vi "LS372Monitor.vi"() -> ()   [LabVIEW 2019]
uses:
  Utility/LS372/LS372-Cluster.ctl
  Instrument_Setup.vi
  Global/Global Variables/Data_Display_global.vi
  Global/Global Variables/global.vi
  Equipment/Lake Shore 372/Lake Shore 372.lvlib
panel:
  out "Tsweeps Running":bool
  out "LS372-Cluster":T1 {"MC Thermometer" items=["Speer 9905", "ROX U02453"]}
  in  "Stopp":bool
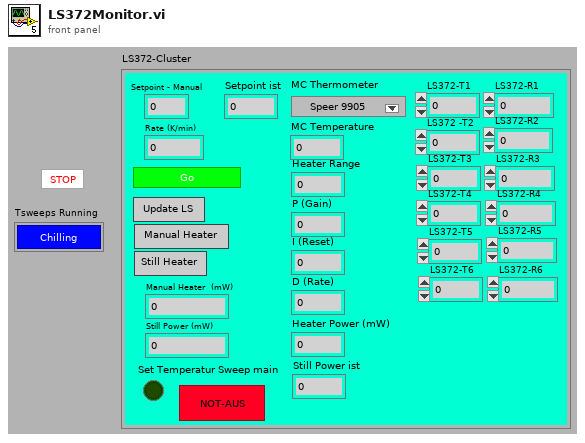
[diagram p1: front panel]
types:
  T1 = typedef "LS372-Cluster.ctl" = cluster{"Activate Tsweep":bool, "Setpoint - Manual":dbl, "Rate (K/min)":dbl, "Update Lakeshores":bool, "Still Heater":bool, "Still Power (mW)":dbl, "Manual Heater":bool, "Manual Heater  (mW) ":dbl, "Heater Range":dbl, "P (Gain)":dbl, "I (Reset)":dbl, "D (Rate)":dbl, "Heater Power (mW)":dbl, "MC Thermometer":u16, "MC Temperature":dbl, "LS372-T1":dbl, "LS372 -T2":dbl, "LS372-R1 ":dbl, "LS372-R2":dbl, "LS372-T3":dbl, "LS372-T4":dbl, "LS372-R3 ":dbl, "LS372-R4 \n\n\n\n":dbl, "LS372-T5":dbl, "LS372-T6":dbl, "LS372-R5":dbl, "LS372-R6 ":dbl, "Still Power ist":dbl, "Set Temperatur Sweep main":bool, "Setpoint ist":dbl, "Disable Heater":bool}
  T2 = typedef "Ls372-Control.ctl" = cluster{"Activate Tsweep":bool, "Setpoint - Manual":dbl, "Rate (K/min)":dbl, "Update Lakeshores":bool, "Still Heater":bool, "Still Power (mW)":dbl, "Manual Heater":bool, "Manual Heater  (mW) ":dbl, "MC Thermometer":u16, "Set Temperature Sweeep main":bool, "Disable Heater":bool}
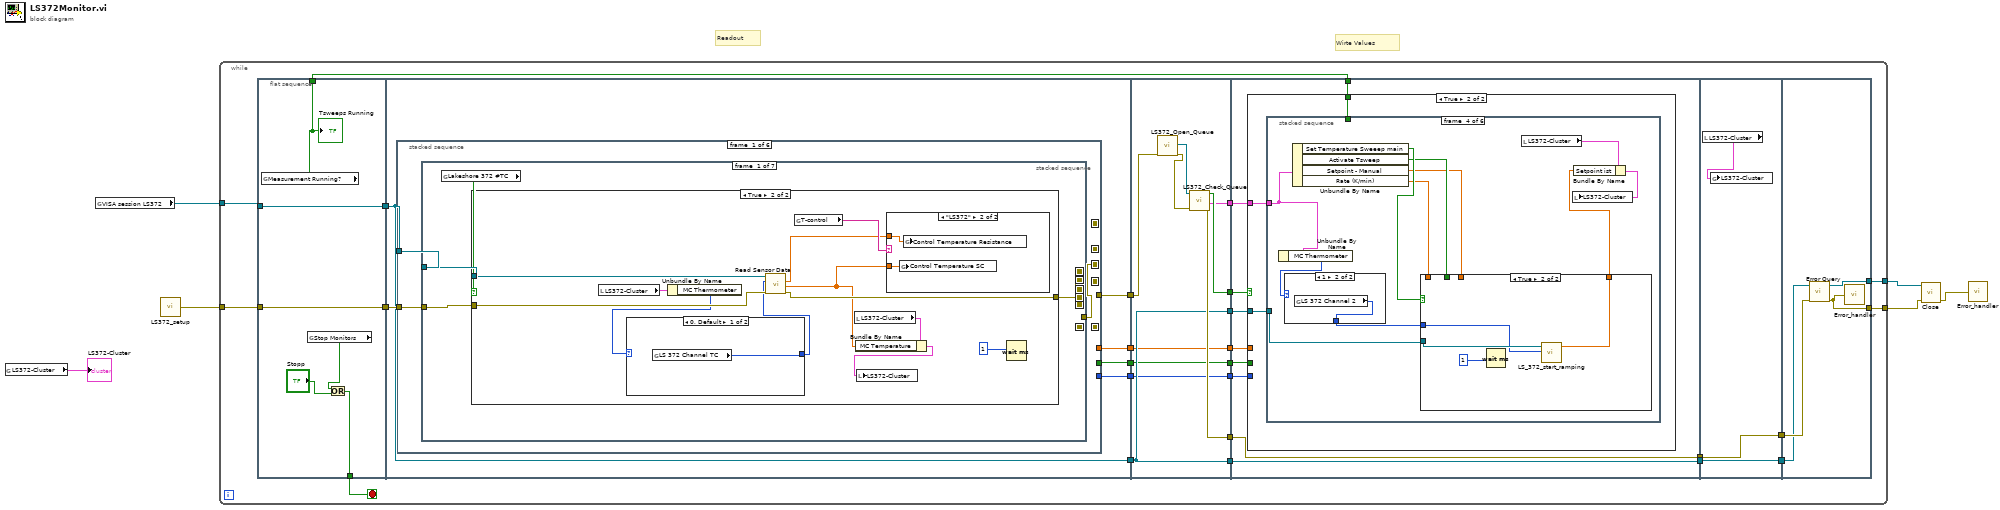
[diagram p0: block diagram]
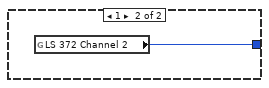
[diagram p3: hidden frame]
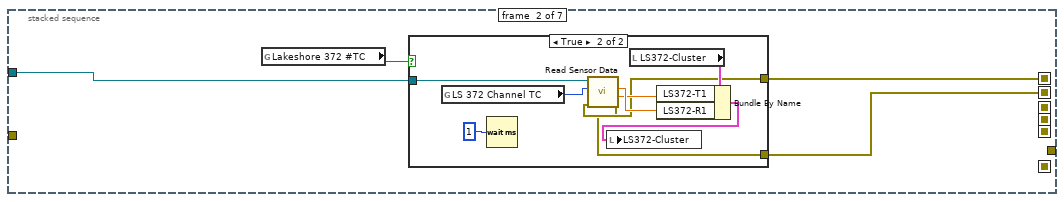
[diagram p5: hidden frame]
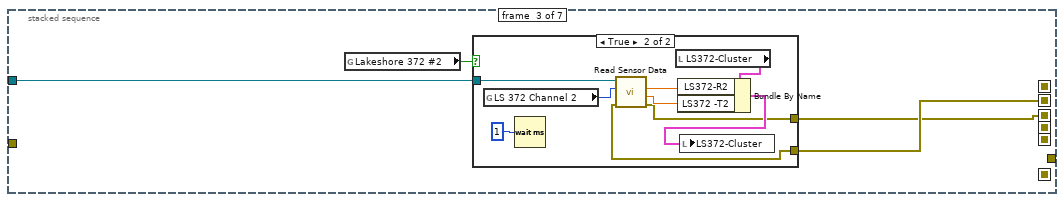
[diagram p7: hidden frame]
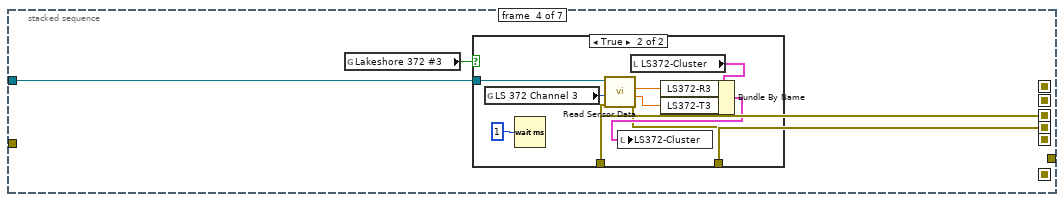
[diagram p9: hidden frame]
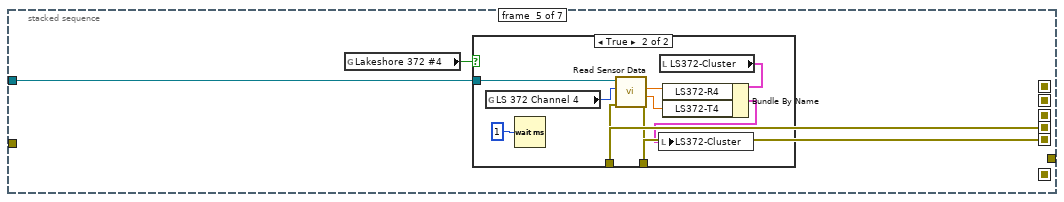
[diagram p11: hidden frame]
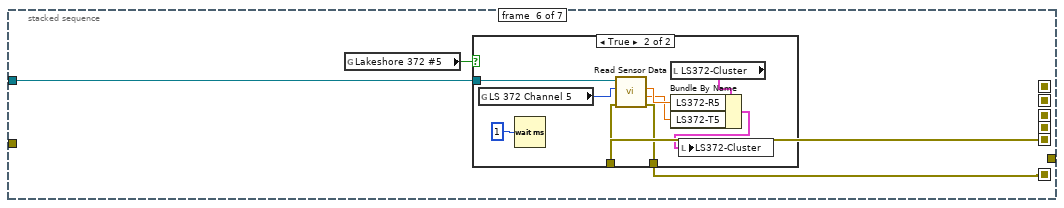
[diagram p13: hidden frame]
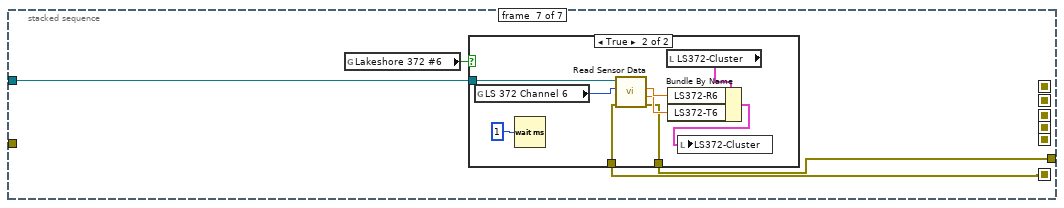
[diagram p15: hidden frame]
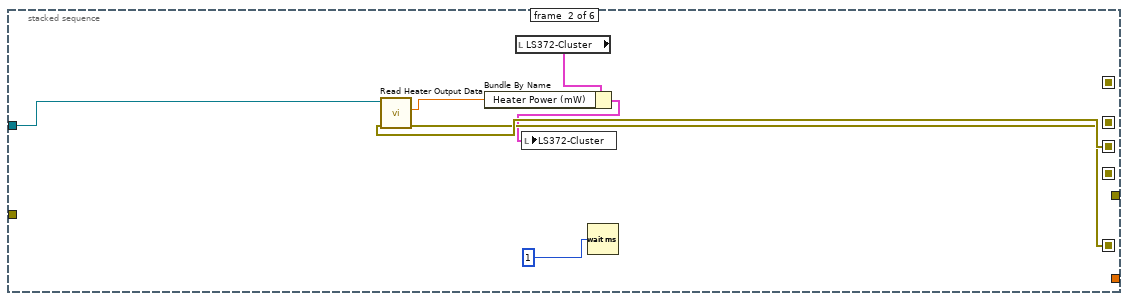
[diagram p17: hidden frame]
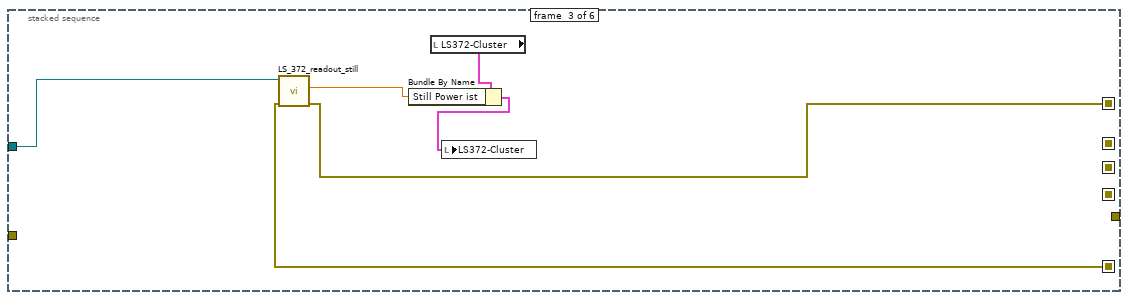
[diagram p18: hidden frame]
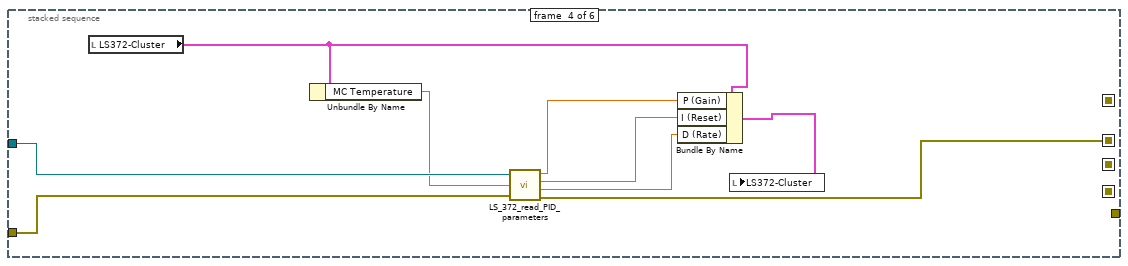
[diagram p19: hidden frame]
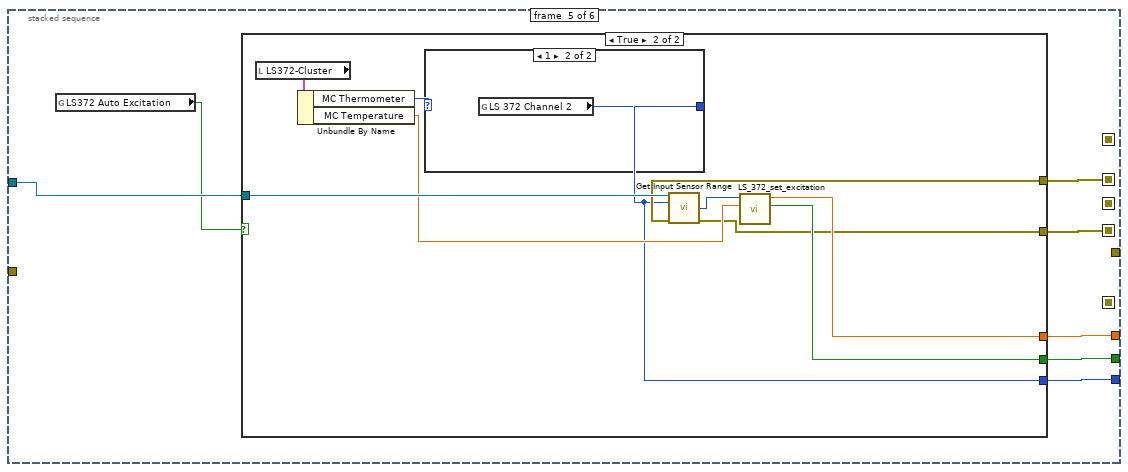
[diagram p20: hidden frame]
diagram:
  # "Wirte Values"
  # "Readout"
  n1 = global read "Data_Display_global.vi" "LS372-Cluster"() -> (→"LS372-Cluster":T1)
  n2 = global read "Instrument_Setup.vi" "VISA session LS372"() -> (w6:refnum<visa-resource-name>)
  n3 = call "LS372_setup.vi"() -> ("error out"=w4:errorcluster)
  n4 = while {
    tunnel: w6 -> [w31]
    tunnel: w4 -> [w25]
    tunnel: [w14] -> w3
    tunnel: [w13] -> w2
    stop <- w29 stop-if-true
    n5 = flat-sequence {
      tunnel: w31 -> [w35]
      tunnel: [w35] -> w30
      tunnel: [w32] -> w29
      tunnel: w25 -> [w34]
      tunnel: [w34] -> w24
      tunnel: [w33] -> w21
      tunnel: w30 -> [w41]
      tunnel: [w42] -> w28
      tunnel: w24 -> [w43]
      tunnel: [w41] -> w23
      tunnel: [w40] -> w11
      tunnel: [w39] -> w9
      tunnel: [w38] -> w7
      tunnel: w28 -> [w212]
      tunnel: [w209] -> w27
      tunnel: [w208] -> w26
      tunnel: w23 -> [w206]
      tunnel: [w206] -> w22
      tunnel: [w207] -> w19
      tunnel: [w206] -> w15
      tunnel: [w205] -> w12
      tunnel: w11 -> [w205]
      tunnel: [w204] -> w10
      tunnel: w9 -> [w204]
      tunnel: [w203] -> w8
      tunnel: w7 -> [w203]
      tunnel: w27 -> [w221]
      tunnel: w26 -> [w220]
      tunnel: w22 -> [w219]
      tunnel: w21 -> [w218]
      tunnel: [w217] -> w20
      tunnel: w19 -> [w217]
      tunnel: [w216] -> w16
      tunnel: w15 -> [w216]
      tunnel: w12 -> [w215]
      tunnel: w10 -> [w214]
      tunnel: w8 -> [w213]
      tunnel: w20 -> [w322]
      tunnel: [w322] -> w18
      tunnel: [w321] -> w17
      tunnel: w16 -> [w321]
      tunnel: w18 -> [w327]
      tunnel: w17 -> [w326]
      tunnel: [w325] -> w14
      tunnel: [w324] -> w13
      frame #0 {
        n6 = global read "global.vi" "Measurement Running?"() -> (w33:bool)
        "Tsweeps Running" <- w33
        n7 = global read "Data_Display_global.vi" "Stop Monitors"() -> (w36:bool)
        n8 = Or(x=w36, y="Stopp") -> (x .or. y?=w32:bool)
      }
      frame #1 {
        n9 = stacked-sequence {
          seq-local: [w44 _ _ _ _ _] -> [_ w156 _ _ _ _]
          seq-local: [_ w155 _ _ _ _] -> [_ _ w163 _ _ _]
          seq-local: [_ _ w162 _ _ _] -> [_ _ _ _ _ _]
          seq-local: [_ _ _ w171 _ _] -> [_ _ _ _ w179 _]
          seq-local: [_ _ _ _ w175 _] -> [_ _ _ _ _ w201]
          tunnel: w41 -> [w46 w158 w164 w173 w180 w202]
          tunnel: w43 -> [w45 _ _ w172 _ _]
          tunnel: [_ _ _ _ _ w200] -> w42
          tunnel: [_ _ _ _ w178 _] -> w40
          tunnel: [_ _ _ _ w177 _] -> w39
          tunnel: [_ _ _ _ w176 _] -> w38
          frame #0 {
            n10 = stacked-sequence {
              seq-local: [w48 _ _ _ _ _ _] -> [_ w69 _ _ _ _ _]
              seq-local: [_ w68 _ _ _ _ _] -> [_ _ w83 _ _ _ _]
              seq-local: [_ _ w82 _ _ _ _] -> [_ _ _ w97 _ _ _]
              seq-local: [_ _ _ w96 _ _ _] -> [_ _ _ _ w111 _ _]
              seq-local: [_ _ _ _ w110 _ _] -> [_ _ _ _ _ w125 _]
              seq-local: [_ _ _ _ _ w124 _] -> [_ _ _ _ _ _ w139]
              tunnel: w46 -> [w50 w70 w84 w98 w112 w126 w140]
              tunnel: w45 -> [w47 _ _ _ _ _ _]
              tunnel: [_ _ _ _ _ _ w138] -> w44
              frame #0 {
                n11 = global read "Instrument_Setup.vi" "Lakeshore 372 #TC"() -> (w49:bool)
                n12 = case shown="True" w49 {
                  tunnel: w50 -> [_ w63]
                  tunnel: [w51 w62] -> w48
                  tunnel: w47 -> [w51 w61]
                  frame False {
                  }
                  frame True {
                    n13 = local read "LS372-Cluster"() -> (w55:T1)
                    n14 = Unbundle By Name(w55) -> ("MC Thermometer"=w54:u16)
                    n15 = case shown="0, Default" w54 {
                      tunnel: [w64 w65] -> w53
                      frame 0, Default {
                        n16 = global read "Instrument_Setup.vi" "LS 372 Channel TC"() -> (w64:u16)
                      }
                      frame 1 {
                        n17 = global read "Instrument_Setup.vi" "LS 372 Channel 2"() -> (w65:u16)
                      }
                    }
                    n18 = call "Read Sensor Data.vi"("error in (no error)"=w61, "Channel (1:1)"=w53, "VISA resource name"=w63) -> ("error out"=w62:errorcluster, "Kelvin Reading"=w57:dbl, "Resistance Reading"=w59:dbl)  [unwired: 3 in, 3 out]
                    n19 = global read "Instrument_Setup.vi" "T-control"() -> (w60:string)
                    n20 = local read "LS372-Cluster"() -> (w58:T1)
                    n21 = Bundle By Name(cluster=w58, "MC Temperature"=w57) -> (w56:T1)
                    n22 = local write "LS372-Cluster"(w56) -> ()
                    n23 = case shown="\"LS372\"" w60 {
                      tunnel: w59 -> [_ w67]
                      tunnel: w57 -> [_ w66]
                      frame "None", Default {
                      }
                      frame "LS372" {
                        n24 = global write "Data_Display_global.vi" "Control Temperature SC"(w66) -> ()
                        n25 = global write "Data_Display_global.vi" "Control Temperature Resistance"(w67) -> ()
                      }
                    }
                    n26 = Wait (ms)(milliseconds to wait=1) -> ()  [unwired: 1 out]
                  }
                }
              }
              frame #1 {
                n27 = global read "Instrument_Setup.vi" "Lakeshore 372 #TC"() -> (w71:bool)
                n28 = case shown="True" w71 {
                  tunnel: w70 -> [_ w80]
                  tunnel: w69 -> [w72 w74]
                  tunnel: [w72 w73] -> w68
                  frame False {
                  }
                  frame True {
                    n29 = global read "Instrument_Setup.vi" "LS 372 Channel TC"() -> (w79:u16)
                    n30 = Wait (ms)(milliseconds to wait=1) -> ()  [unwired: 1 out]
                    n31 = call "Read Sensor Data.vi"("error in (no error)"=w74, "Channel (1:1)"=w79, "VISA resource name"=w80) -> ("error out"=w73:errorcluster, "Kelvin Reading"=w75:dbl, "Resistance Reading"=w76:dbl)  [unwired: 3 in, 3 out]
                    n32 = local read "LS372-Cluster"() -> (w78:T1)
                    n33 = Bundle By Name(cluster=w78, "LS372-T1"=w75, "LS372-R1"=w76) -> (w77:T1)
                    n34 = local write "LS372-Cluster"(w77) -> ()
                  }
                }
              }
              frame #2 {
                n35 = global read "Instrument_Setup.vi" "Lakeshore 372 #2"() -> (w85:bool)
                n36 = case shown="True" w85 {
                  tunnel: w84 -> [_ w94]
                  tunnel: w83 -> [w86 w88]
                  tunnel: [w86 w87] -> w82
                  frame False {
                  }
                  frame True {
                    n37 = global read "Instrument_Setup.vi" "LS 372 Channel 2"() -> (w93:u16)
                    n38 = Wait (ms)(milliseconds to wait=1) -> ()  [unwired: 1 out]
                    n39 = call "Read Sensor Data.vi"("error in (no error)"=w88, "Channel (1:1)"=w93, "VISA resource name"=w94) -> ("error out"=w87:errorcluster, "Kelvin Reading"=w89:dbl, "Resistance Reading"=w90:dbl)  [unwired: 3 in, 3 out]
                    n40 = local read "LS372-Cluster"() -> (w92:T1)
                    n41 = Bundle By Name(cluster=w92, "LS372-R2"=w90, "LS372 -T2"=w89) -> (w91:T1)
                    n42 = local write "LS372-Cluster"(w91) -> ()
                  }
                }
              }
              frame #3 {
                n43 = global read "Instrument_Setup.vi" "Lakeshore 372 #3"() -> (w99:bool)
                n44 = case shown="True" w99 {
                  tunnel: w98 -> [_ w108]
                  tunnel: w97 -> [w100 w102]
                  tunnel: [w100 w101] -> w96
                  frame False {
                  }
                  frame True {
                    n45 = global read "Instrument_Setup.vi" "LS 372 Channel 3"() -> (w107:u16)
                    n46 = Wait (ms)(milliseconds to wait=1) -> ()  [unwired: 1 out]
                    n47 = call "Read Sensor Data.vi"("error in (no error)"=w102, "Channel (1:1)"=w107, "VISA resource name"=w108) -> ("error out"=w101:errorcluster, "Kelvin Reading"=w103:dbl, "Resistance Reading"=w104:dbl)  [unwired: 3 in, 3 out]
                    n48 = local read "LS372-Cluster"() -> (w106:T1)
                    n49 = Bundle By Name(cluster=w106, "LS372-R3"=w104, "LS372-T3"=w103) -> (w105:T1)
                    n50 = local write "LS372-Cluster"(w105) -> ()
                  }
                }
              }
              frame #4 {
                n51 = global read "Instrument_Setup.vi" "Lakeshore 372 #4"() -> (w113:bool)
                n52 = case shown="True" w113 {
                  tunnel: w112 -> [_ w122]
                  tunnel: w111 -> [w114 w116]
                  tunnel: [w114 w115] -> w110
                  frame False {
                  }
                  frame True {
                    n53 = global read "Instrument_Setup.vi" "LS 372 Channel 4"() -> (w121:u16)
                    n54 = Wait (ms)(milliseconds to wait=1) -> ()  [unwired: 1 out]
                    n55 = call "Read Sensor Data.vi"("error in (no error)"=w116, "Channel (1:1)"=w121, "VISA resource name"=w122) -> ("error out"=w115:errorcluster, "Kelvin Reading"=w117:dbl, "Resistance Reading"=w118:dbl)  [unwired: 3 in, 3 out]
                    n56 = local read "LS372-Cluster"() -> (w120:T1)
                    n57 = Bundle By Name(cluster=w120, "LS372-R4"=w118, "LS372-T4"=w117) -> (w119:T1)
                    n58 = local write "LS372-Cluster"(w119) -> ()
                  }
                }
              }
              frame #5 {
                n59 = global read "Instrument_Setup.vi" "Lakeshore 372 #5"() -> (w127:bool)
                n60 = case shown="True" w127 {
                  tunnel: w126 -> [_ w136]
                  tunnel: w125 -> [w128 w130]
                  tunnel: [w128 w129] -> w124
                  frame False {
                  }
                  frame True {
                    n61 = global read "Instrument_Setup.vi" "LS 372 Channel 5"() -> (w135:u16)
                    n62 = Wait (ms)(milliseconds to wait=1) -> ()  [unwired: 1 out]
                    n63 = call "Read Sensor Data.vi"("error in (no error)"=w130, "Channel (1:1)"=w135, "VISA resource name"=w136) -> ("error out"=w129:errorcluster, "Kelvin Reading"=w131:dbl, "Resistance Reading"=w132:dbl)  [unwired: 3 in, 3 out]
                    n64 = local read "LS372-Cluster"() -> (w134:T1)
                    n65 = Bundle By Name(cluster=w134, "LS372-R5"=w132, "LS372-T5"=w131) -> (w133:T1)
                    n66 = local write "LS372-Cluster"(w133) -> ()
                  }
                }
              }
              frame #6 {
                n67 = global read "Instrument_Setup.vi" "Lakeshore 372 #6"() -> (w141:bool)
                n68 = case shown="True" w141 {
                  tunnel: w140 -> [_ w150]
                  tunnel: w139 -> [w142 w144]
                  tunnel: [w142 w143] -> w138
                  frame False {
                  }
                  frame True {
                    n69 = global read "Instrument_Setup.vi" "LS 372 Channel 6"() -> (w149:u16)
                    n70 = Wait (ms)(milliseconds to wait=1) -> ()  [unwired: 1 out]
                    n71 = call "Read Sensor Data.vi"("error in (no error)"=w144, "Channel (1:1)"=w149, "VISA resource name"=w150) -> ("error out"=w143:errorcluster, "Kelvin Reading"=w145:dbl, "Resistance Reading"=w146:dbl)  [unwired: 3 in, 3 out]
                    n72 = local read "LS372-Cluster"() -> (w148:T1)
                    n73 = Bundle By Name(cluster=w148, "LS372-R6"=w146, "LS372-T6"=w145) -> (w147:T1)
                    n74 = local write "LS372-Cluster"(w147) -> ()
                  }
                }
              }
            }
          }
          frame #1 {
            n75 = call "Read Heater Output Data.vi"("error in (no error)"=w156, "VISA resource name"=w158) -> ("error out"=w155:errorcluster, "Heater Output"=w152:dbl)  [unwired: 7 in, 1 out]
            n76 = local read "LS372-Cluster"() -> (w154:T1)
            n77 = Bundle By Name(cluster=w154, "Heater Power (mW)"=w152) -> (w153:T1)
            n78 = local write "LS372-Cluster"(w153) -> ()
            n79 = Wait (ms)(milliseconds to wait=1) -> ()  [unwired: 1 out]
          }
          frame #2 {
            n80 = call "LS_372_readout_still.vi"("error in (no error)"=w163, "VISA-Ressourcenname (in)"=w164) -> ("error out"=w162:errorcluster, "Still Value"=w159:dbl)  [unwired: 3 in, 1 out]
            n81 = local read "LS372-Cluster"() -> (w161:T1)
            n82 = Bundle By Name(cluster=w161, "Still Power ist"=w159) -> (w160:T1)
            n83 = local write "LS372-Cluster"(w160) -> ()
          }
          frame #3 {
            n84 = local read "LS372-Cluster"() -> (w166:T1)
            n85 = Unbundle By Name(w166) -> ("MC Temperature"=w165:dbl)
            n86 = call "LS_372_read_PID_parameters.vi"("VISA-Ressourcenname (in)"=w173, "Temperature"=w165, "error in (no error)"=w172) -> ("Gain (P)"=w169:dbl, "Reset (I)"=w168:dbl, "Rate (D)"=w167:dbl, "error out"=w171:errorcluster)  [unwired: 1 out]
            n87 = Bundle By Name(cluster=w166, "P (Gain)"=w169, "I (Reset)"=w168, "D (Rate)"=w167) -> (w170:T1)
            n88 = local write "LS372-Cluster"(w170) -> ()
          }
          frame #4 {
            n89 = global read "Instrument_Setup.vi" "LS372 Auto Excitation"() -> (w174:bool)
            n90 = case shown="True" w174 {
              tunnel: w180 -> [_ w194]
              tunnel: w179 -> [w184 w193]
              tunnel: [5.0 w188] -> w178
              tunnel: [FALSE w187] -> w177
              tunnel: [1 w186] -> w176
              tunnel: [w184 w185] -> w175
              frame False {
              }
              frame True {
                n91 = local read "LS372-Cluster"() -> (w192:T1)
                n92 = Unbundle By Name(w192) -> ("MC Thermometer"=w191:u16, "MC Temperature"=w189:dbl)
                n93 = case shown="1" w191 {
                  tunnel: [w195 w196] -> w186
                  frame 0, Default {
                    n94 = global read "Instrument_Setup.vi" "LS 372 Channel TC"() -> (w195:u16)
                  }
                  frame 1 {
                    n95 = global read "Instrument_Setup.vi" "LS 372 Channel 2"() -> (w196:u16)
                  }
                }
                n96 = call "Get Input Sensor Range.vi"("VISA resource name"=w194, "Channel (1:1)"=w186, "error in (no error)"=w193) -> ("Excitation Range"=w190:u16, "error out"=w185:errorcluster)  [unwired: 5 in, 6 out]
                n97 = call "LS_372_set_excitation.vi"("Temperature"=w189, "LS_Excitation old"=w190) -> ("Change of Excitation?"=w187:bool, "LS_Excitation new"=w188:dbl)  [unwired: 4 in]
              }
            }
          }
          frame #5 {
            n98 = call "LS_372_read_heater_range.vi"("Error In"=w201, "VISA (in)"=w202) -> ("Error Out"=w200:errorcluster, "Numeric"=w197:dbl)  [unwired: 1 in, 1 out]
            n99 = local read "LS372-Cluster"() -> (w199:T1)
            n100 = Bundle By Name(cluster=w199, "Heater Range"=w197) -> (w198:T1)
            n101 = local write "LS372-Cluster"(w198) -> ()
          }
        }
      }
      frame #2 {
        n102 = call "LS372_Open_Queue.vi"("error in (no error)"=w212) -> ("error out"=w211:errorcluster, "queue out"=w210:refnum<queue>)  [unwired: 9 in]
        n103 = call "LS372_Check_Queue.vi"("error in (no error)"=w211, "queue"=w210) -> ("error out"=w207:errorcluster, "LS372-Control"=w208:T2, "New Entries?"=w209:bool)  [unwired: 6 in]
      }
      frame #3 {
        n104 = case shown="True" w221 {
          tunnel: w220 -> [_ w233]
          tunnel: w219 -> [w225 w232]
          tunnel: w218 -> [_ w231]
          tunnel: w215 -> [w224 _]
          tunnel: w214 -> [w222 _]
          tunnel: w213 -> [w223 _]
          frame False {
            n105 = case shown="True" w222 {
              tunnel: w225 -> [_ w230]
              tunnel: w224 -> [_ w229]
              tunnel: w223 -> [_ w228]
              frame False {
              }
              frame True {
                n106 = call "Configure Input Sensor Range.vi"("VISA resource name"=w230, "Channel (1)"=w228, "Excitation Range (5: 200 uV / 100 pA)"=w229, "Autorange (0: Autorange off)"=1, "Preferred Units (2: Ohms)"=1) -> ()  [unwired: 13 in, 2 out]
              }
            }
          }
          frame True {
            n107 = stacked-sequence {
              tunnel: w233 -> [w238 w255 w263 w268 w301 w320]
              tunnel: w232 -> [w236 w253 w256 w276 w302 _]
              tunnel: w231 -> [_ _ w262 _ _ _]
              frame #0 {
                n108 = Unbundle By Name(w238) -> ("Update Lakeshores"=w237:bool, "MC Thermometer"=w235:u16)
                n109 = case shown="1" w235 {
                  tunnel: [w239 w240] -> w234
                  frame 0, Default {
                    n110 = global read "Instrument_Setup.vi" "LS 372 Channel TC"() -> (w239:u16)
                  }
                  frame 1 {
                    n111 = global read "Instrument_Setup.vi" "LS 372 Channel 2"() -> (w240:u16)
                  }
                }
                n112 = case shown="True" w237 {
                  tunnel: w236 -> [_ w243]
                  tunnel: w234 -> [_ w241]
                  frame False {
                  }
                  frame True {
                    n113 = flat-sequence {
                      tunnel: [w246] -> w244
                      tunnel: w243 -> [w246]
                      tunnel: [w245] -> w242
                      tunnel: w241 -> [w245]
                      tunnel: w244 -> [w249]
                      tunnel: w242 -> [w248]
                      frame #0 {
                        n114 = call "LS372_setup.vi"() -> ()  [unwired: 1 out]
                        n115 = Wait (ms)(milliseconds to wait=50) -> ()  [unwired: 1 out]
                      }
                      frame #1 {
                        n116 = call "LS372_set_main_measuring_channel.vi"("VISA resource name"=w249, "Channel"=w248) -> ()  [unwired: 4 in, 1 out]
                      }
                    }
                  }
                }
              }
              frame #1 {
                # "Set Still Power"
                n117 = global read "Instrument_Setup.vi" "LS 372  Still Heater Resistance"() -> (w250:dbl)
                n118 = Unbundle By Name(w255) -> ("Still Heater"=w252:bool, "Still Power (mW)"=w251:dbl)
                n119 = call "LS_372_still_control.vi"("Still Resistance"=w250, "Still Power"=w251, "Still heater"=w252, "VISA-Ressourcenname"=w253) -> ()  [unwired: 4 in]
                n120 = Wait (ms)(milliseconds to wait=1) -> ()  [unwired: 1 out]
              }
              frame #2 {
                # "Set Heater Power manuel"
                n121 = Unbundle By Name(w263) -> ("Manual Heater  (mW)"=w258:dbl, "Manual Heater"=w260:bool)
                n122 = Not(x=w262) -> (.not. x?=w261:bool)
                n123 = And(x=w261, y=w260) -> (x .and. y?=w259:bool)
                n124 = case shown="True" w259 {
                  selector: w259 -> [_ w267]
                  tunnel: w258 -> [_ w266]
                  tunnel: w256 -> [_ w264]
                  frame False {
                  }
                  frame True {
                    n125 = global read "Instrument_Setup.vi" "LS 372 MC Heater Resistance"() -> (w265:dbl)
                    n126 = call "LS372_manual_heater_output.vi"("Heater Resistance"=w265, "Heater Power"=w266, "Manuel Heater"=w267, "VISA-Ressourcenname"=w264) -> ()  [unwired: 4 in]
                  }
                }
                n127 = Wait (ms)(milliseconds to wait=1) -> ()  [unwired: 1 out]
              }
              frame #3 {
                n128 = Unbundle By Name(w268) -> ("MC Thermometer"=w269:u16)
                n129 = case shown="1" w269 {
                  tunnel: [w279 w280] -> w270
                  frame 0, Default {
                    n130 = global read "Instrument_Setup.vi" "LS 372 Channel TC"() -> (w279:u16)
                  }
                  frame 1 {
                    n131 = global read "Instrument_Setup.vi" "LS 372 Channel 2"() -> (w280:u16)
                  }
                }
                n132 = Unbundle By Name(w268) -> ("Set Temperature Sweeep main"=w278:bool, "Activate Tsweep"=w277:bool, "Setpoint - Manual"=w272:dbl, "Rate (K/min)"=w271:dbl)
                n133 = case shown="True" w278 {
                  tunnel: w277 -> [w286 _]
                  tunnel: w276 -> [w282 w299]
                  tunnel: [w281 w298] -> w273
                  tunnel: w272 -> [w284 _]
                  tunnel: w271 -> [w285 _]
                  tunnel: w270 -> [w283 w297]
                  frame False {
                    n134 = case shown="True" w286 {
                      tunnel: w285 -> [_ w296]
                      tunnel: w284 -> [_ w293]
                      tunnel: w283 -> [_ w295]
                      tunnel: w282 -> [_ w294]
                      tunnel: [w287 w293] -> w281
                      frame False {
                        n135 = global read "global.vi" "Cerrent State"() -> (w290:i32)
                        n136 = Equal?(x=1, y=w290) -> (x = y?=w288:bool)
                        n137 = case shown="False" w288 {
                          tunnel: [w291 w292] -> w287
                          frame False {
                            n138 = global read "global.vi" "T final (K)"() -> (w291:dbl)
                          }
                          frame True {
                            n139 = global read "global.vi" "T init. (K)"() -> (w292:dbl)
                          }
                        }
                      }
                      frame True {
                        n140 = call "LS_372_manual_ramping.vi"("Setpoint"=w293, "Rate"=w296, "Channel"=w295, "VISA-Ressourcenname"=w294) -> ()  [unwired: 4 in]
                      }
                    }
                  }
                  frame True {
                    n141 = Wait (ms)(milliseconds to wait=1) -> ()  [unwired: 1 out]
                    n142 = call "LS_372_start_ramping.vi"("Channel"=w297, "VISA-Ressourcenname"=w299) -> ("Setpoint"=w298:dbl)  [unwired: 5 in]
                  }
                }
                n143 = local read "LS372-Cluster"() -> (w275:T1)
                n144 = Bundle By Name(cluster=w275, "Setpoint ist"=w273) -> (w274:T1)
                n145 = local write "LS372-Cluster"(w274) -> ()
              }
              frame #4 {
                n146 = Unbundle By Name(w301) -> ("Disable Heater"=w303:bool)
                n147 = case shown="True" w303 {
                  tunnel: w302 -> [_ w305]
                  tunnel: w301 -> [_ w304]
                  frame False {
                  }
                  frame True {
                    n148 = Unbundle By Name(w304) -> ("MC Thermometer"=w309:u16)
                    n149 = case shown="0, Default" w309 {
                      tunnel: [w312 w315] -> w306
                      tunnel: w305 -> [w311 w314]
                      frame 0, Default {
                        n150 = global read "Instrument_Setup.vi" "LS 372 Channel TC"() -> (w313:u16)
                        n151 = call "LS_372_disable_heater.vi"("Channel"=w313, "VISA-Ressourcenname"=w311) -> ("Setpoint ist"=w312:dbl)  [unwired: 5 in]
                      }
                      frame 1 {
                        n152 = global read "Instrument_Setup.vi" "LS 372 Channel 2"() -> (w316:u16)
                        n153 = call "LS_372_disable_heater.vi"("Channel"=w316, "VISA-Ressourcenname"=w314) -> ("Setpoint ist"=w315:dbl)  [unwired: 5 in]
                      }
                    }
                    n154 = local read "LS372-Cluster"() -> (w308:T1)
                    n155 = Bundle By Name(cluster=w308, "Setpoint ist"=w306) -> (w307:T1)
                    n156 = local write "LS372-Cluster"(w307) -> ()
                    n157 = Wait (ms)(milliseconds to wait=10) -> ()  [unwired: 1 out]
                  }
                }
              }
              frame #5 {
                n158 = Unbundle By Name(w320) -> ("MC Thermometer"=w318:u16)
                n159 = local read "LS372-Cluster"() -> (w319:T1)
                n160 = Bundle By Name(cluster=w319, "MC Thermometer"=w318) -> (w317:T1)
                n161 = local write "LS372-Cluster"(w317) -> ()
              }
            }
          }
        }
      }
      frame #4 {
        n162 = local read "LS372-Cluster"() -> (w323:T1)
        n163 = global write "Data_Display_global.vi" "LS372-Cluster"(w323) -> ()
      }
      frame #5 {
        n164 = call "Error Query.vi"("error in (no error)"=w327, "VISA resource name"=w326) -> ("error out"=w325:errorcluster, "VISA resource name out"=w324:refnum<visa-resource-name>)  [unwired: 7 in, 1 out]
        n165 = call "Error_handler.vi"("error constant"=w325) -> ()
      }
    }
  }
  n166 = call "Close.vi"("error in (no error)"=w3, "VISA resource name"=w2) -> ("error out"=w1:errorcluster)  [unwired: 9 in]
  n167 = call "Error_handler.vi"("error constant"=w1) -> ()
